vi "AAP.vi"() -> ()   [LabVIEW 2014]
panel:
  out "Average Value":dbl
  out "Waveform Graph":dynamicdata(graph)
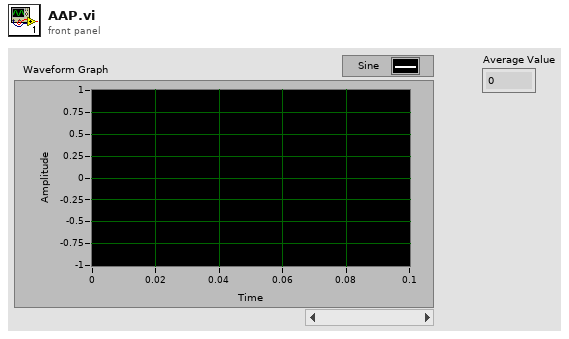
[diagram p1: front panel]
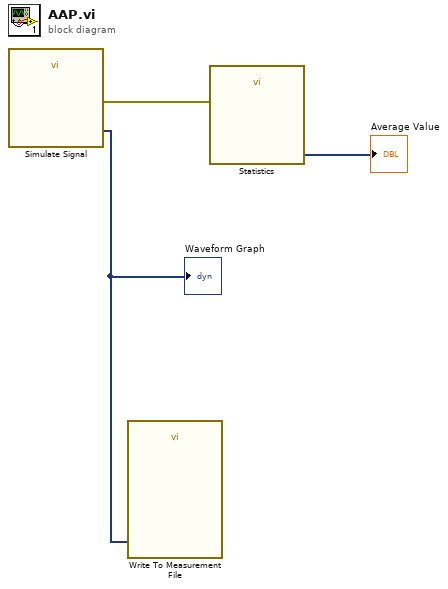
[diagram p0: block diagram]
diagram:
  n1 = call "Simulate Signal"() -> ("Sine"=w1:dynamicdata, "error out"=w3:errorcluster)  [unwired: 14 in]
  "Waveform Graph" <- w1
  n2 = call "Write To Measurement File"("Signals"=w1) -> ()  [unwired: 16 in, 3 out]
  n3 = call "Statistics"("error in (no error)"=w3) -> ("Arithmetic Mean"=→"Average Value":dynamicdata)  [unwired: 25 in, 1 out]
